vi "Add Menu Measurement.vi"(8 "error in (no error)":errorcluster, 10 "Name":string, 11 "Common Measurements Interface in":refnum<class "Common Measurements Interface.lvclass">) -> (0 "error out":errorcluster, 3 "Common Measurements Interface out":refnum<class "Common Measurements Interface.lvclass">)   [LabVIEW 2015, in "Common Measurements Interface.lvclass"]
uses:
  Common Measurements Interface.lvclass
  Common Measurements Interface.lvclass/Common Measurements Interface.ctl
  Queued Listbox/Queued Listbox.xctl
  Mag Lab Error Handler/Mag Lab Error Handler.lvclass
panel:
  out "Current Strings":string[](array[string])
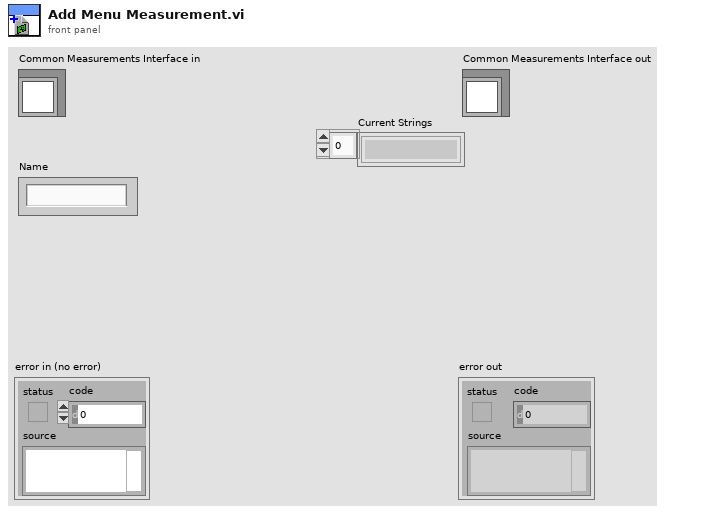
[diagram p1: front panel]
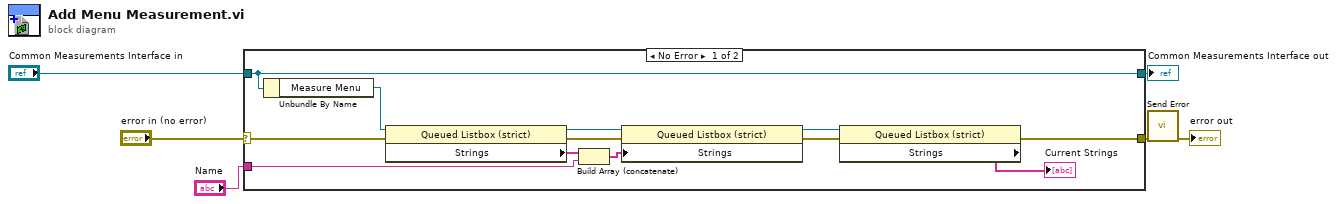
[diagram p0: block diagram]
diagram:
  n1 = case shown="No Error" "error in (no error)" {
    selector: "error in (no error)" -> [w14 w20]
    tunnel: [w8 w20] -> w5
    tunnel: [w18 w19] -> w3
    tunnel: "Common Measurements Interface in" -> [w18 w19]
    tunnel: "Name" -> [w15 _]
    frame No Error {
      n2 = Unbundle By Name(w18) -> ("Measure Menu"=w11:refnum<vi>)
      n3 = property class="Queued Listbox (strict)"(reference=w11, error in=w14) -> (reference out=w17:refnum<vi>, error out=w13:errorcluster, "Strings"=w16:string[])
      n4 = Build Array (concatenate)(w16, w15) -> (w12:string[])
      n5 = property class="Queued Listbox (strict)"(reference=w17, error in=w13, "Strings"=w12) -> (reference out=w9:refnum<vi>, error out=w10:errorcluster)
      n6 = property class="Queued Listbox (strict)"(reference=w9, error in=w10) -> (error out=w8:errorcluster, "Strings"=→"Current Strings":string[])  [unwired: 1 out]
    }
    frame Error {
    }
  }
  "Common Measurements Interface out" <- w3
  n7 = call "Send Error.vi"("error in (no error)"=w5) -> ("error out"=→"error out":errorcluster)  [unwired: 9 in, 1 out]
